vi "Fixed Counter with FGV.vi"() -> ()   [LabVIEW 2012]
uses:
  Up Down Counter Command.ctl
panel:
  out "Running Total":i32
  in  "Stop Button":bool
  out "Loop Count Difference":i32
  out "Loop Count 2":i32
  out "Loop Count 1":i32
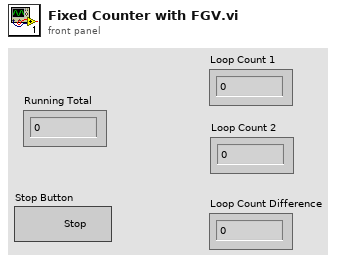
[diagram p1: front panel]
types:
  T1 = typedef "Up Down Counter Command.ctl" = enum16{"Reset", "Increment", "Decrement", "Get Current Value"}
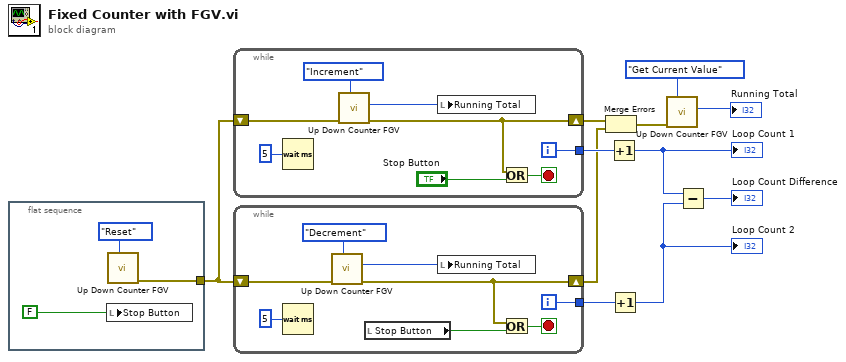
[diagram p0: block diagram]
diagram:
  n1 = flat-sequence {
    tunnel: [w12] -> w3
    frame #0 {
      n2 = local write "Stop Button"(FALSE ("Stop Button")) -> ()
      n3 = call "Up Down Counter FGV.vi"("Action Selection"=Up_Down_Counter_Command."Reset") -> ("Error Out"=w12:errorcluster)  [unwired: 9 in, 1 out]
    }
  }
  n4 = while {
    tunnel: [w20] -> w11
    shift-right: [w15] -> w6
    shift-left: w3 -> [w18]
    i -> [w20]
    stop <- w16 stop-if-true
    n5 = Wait (ms)(milliseconds to wait=u32 5) -> ()  [unwired: 1 out]
    n6 = call "Up Down Counter FGV.vi"("Action Selection"=Up_Down_Counter_Command."Increment", "Error In"=w18) -> ("Error Out"=w15:errorcluster, "Running Total"=w17:i32)  [unwired: 8 in]
    n7 = local write "Running Total"(w17) -> ()
    n8 = Or(x=w15, y="Stop Button") -> (x .or. y?=w16:bool)
  }
  n9 = while {
    tunnel: [w28] -> w10
    shift-right: [w23] -> w1
    shift-left: w3 -> [w25]
    i -> [w28]
    stop <- w24 stop-if-true
    n10 = Wait (ms)(milliseconds to wait=u32 5) -> ()  [unwired: 1 out]
    n11 = call "Up Down Counter FGV.vi"("Action Selection"=Up_Down_Counter_Command."Decrement", "Error In"=w25) -> ("Error Out"=w23:errorcluster, "Running Total"=w27:i32)  [unwired: 8 in]
    n12 = local read "Stop Button"() -> (w30:bool)
    n13 = local write "Running Total"(w27) -> ()
    n14 = Or(x=w23, y=w30) -> (x .or. y?=w24:bool)
  }
  n15 = Merge Errors(w6, w1) -> (w2:errorcluster)
  n16 = Increment(x=w11) -> (x+1=w9:i32)
  "Loop Count 1" <- w9
  n17 = Increment(x=w10) -> (x+1=w8:i32)
  "Loop Count 2" <- w8
  n18 = call "Up Down Counter FGV.vi"("Action Selection"=Up_Down_Counter_Command."Get Current Value", "Error In"=w2) -> ("Running Total"=→"Running Total":i32)  [unwired: 8 in, 1 out]
  n19 = Subtract(x=w9, y=w8) -> (x-y=→"Loop Count Difference":i32)
